vi "Test_of_the_stim_settings_save.vi"() -> ()   [LabVIEW 2016]
panel:
  out "Array 3":T1(array[cluster])
  out "Array 2":string[](array[string])
  out "data string 2":string
  out "value":T2(array[cluster])
  out "data string":string
  out "Array":T2(array[cluster])
  in  "Path to the settings file":path=path "D:/Users/Dmitriy/CData/CloudStation/Tracker_repository/Tracker_settings.tcf"
  in  "Stimulus presets":T1(array[cluster])=[{"Event type"=0, "Cond., s"=0.10000000149011612, "Stim., s"=0.10000000149011612, "Set/Clear"=FALSE, "TTL out N"=1, "Stim. has been set"=TRUE}, {"Event type"=0, "Cond., s"=0.20000000298023224, "Stim., s"=0.20000000298023224, "Set/Clear"=FALSE, "TTL out N"=2, "Stim. has been set"=TRUE}, {"Event type"=0, "Cond., s"=0.0, "Stim., s"=0.0, "Set/Clear"=FALSE, "TTL out N"=1, "Stim. has been set"=FALSE}, {"Event type"=0, "Cond., s"=0.4000000059604645, "Stim., s"=0.4000000059604645, "Set/Clear"=FALSE, "TTL out N"=2, "Stim. has been set"=TRUE}, {"Event type"=0, "Cond., s"=0.0, "Stim., s"=0.0, "Set/Clear"=FALSE, "TTL out N"=1, "Stim. has been set"=FALSE}, {"Event type"=0, "Cond., s"=0.0, "Stim., s"=0.0, "Set/Clear"=FALSE, "TTL out N"=1, "Stim. has been set"=FALSE}, {"Event type"=0, "Cond., s"=0.0, "Stim., s"=0.0, "Set/Clear"=FALSE, "TTL out N"=1, "Stim. has been set"=FALSE}, {"Event type"=0, "Cond., s"=0.0, "Stim., s"=0.0, "Set/Clear"=FALSE, "TTL out N"=1, "Stim. has been set"=FALSE}, {"Event type"=0, "Cond., s"=0.0, "Stim., s"=0.0, "Set/Clear"=FALSE, "TTL out N"=1, "Stim. has been set"=FALSE}, {"Event type"=0, "Cond., s"=0.0, "Stim., s"=0.0, "Set/Clear"=FALSE, "TTL out N"=1, "Stim. has been set"=FALSE}, {"Event type"=0, "Cond., s"=0.0, "Stim., s"=0.0, "Set/Clear"=FALSE, "TTL out N"=1, "Stim. has been set"=FALSE}, {"Event type"=0, "Cond., s"=0.0, "Stim., s"=0.0, "Set/Clear"=FALSE, "TTL out N"=1, "Stim. has been set"=FALSE}, {"Event type"=0, "Cond., s"=0.0, "Stim., s"=0.0, "Set/Clear"=FALSE, "TTL out N"=1, "Stim. has been set"=FALSE}, {"Event type"=0, "Cond., s"=0.0, "Stim., s"=0.0, "Set/Clear"=FALSE, "TTL out N"=1, "Stim. has been set"=FALSE}] {"TTL out N" items=["1"=1, "2"=2]; "Stim., s" min=0.0 max=10000.0 step=0.05000000074505806; "Cond., s" min=0.0 max=10000.0 step=0.05000000074505806 format="%#.2f"; "Event type" items=["Stay for N seconds"]}
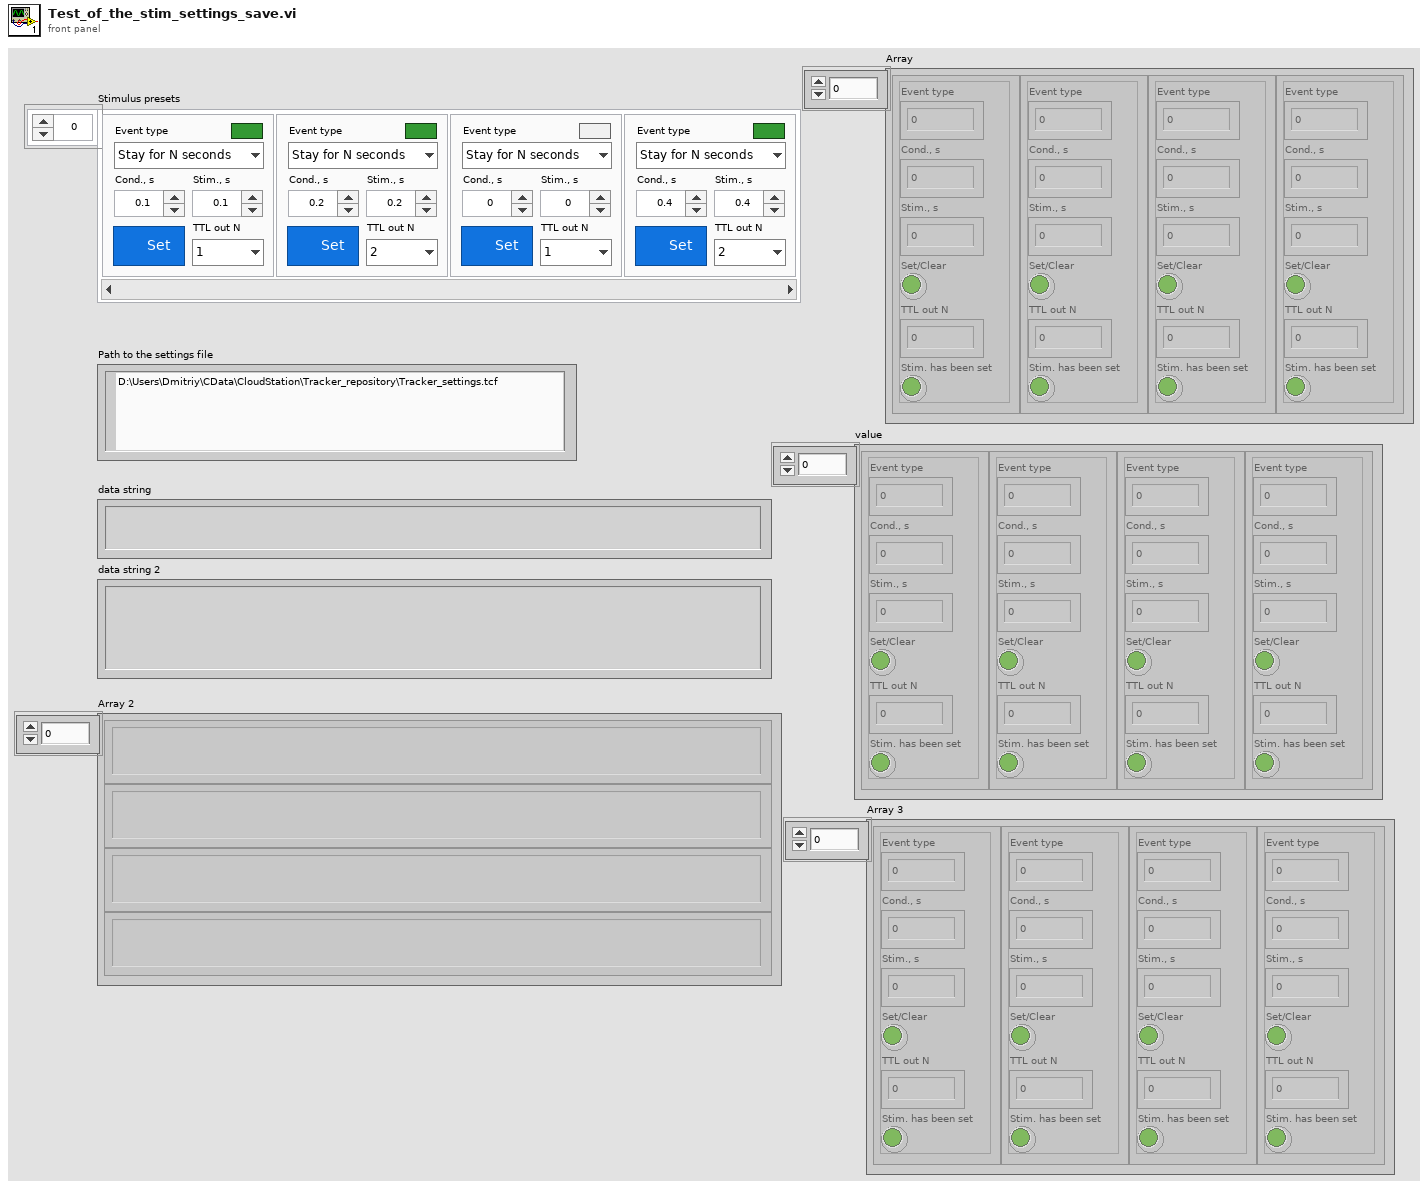
[diagram p1: front panel]
types:
  T1 = cluster{"Event type":u16, "Cond., s":dbl, "Stim., s":dbl, "Set/Clear":bool, "TTL out N":u16, "Stim. has been set":bool}[]
  T2 = cluster{"Event type":u16, "Cond., s":sgl, "Stim., s":sgl, "Set/Clear":bool, "TTL out N":u16, "Stim. has been set":bool}[]
  T3 = cluster{"Event type":u16, "Cond., s":dbl, "Stim., s":dbl, "Set/Clear":bool, "TTL out N":u16, "Stim. has been set":bool}
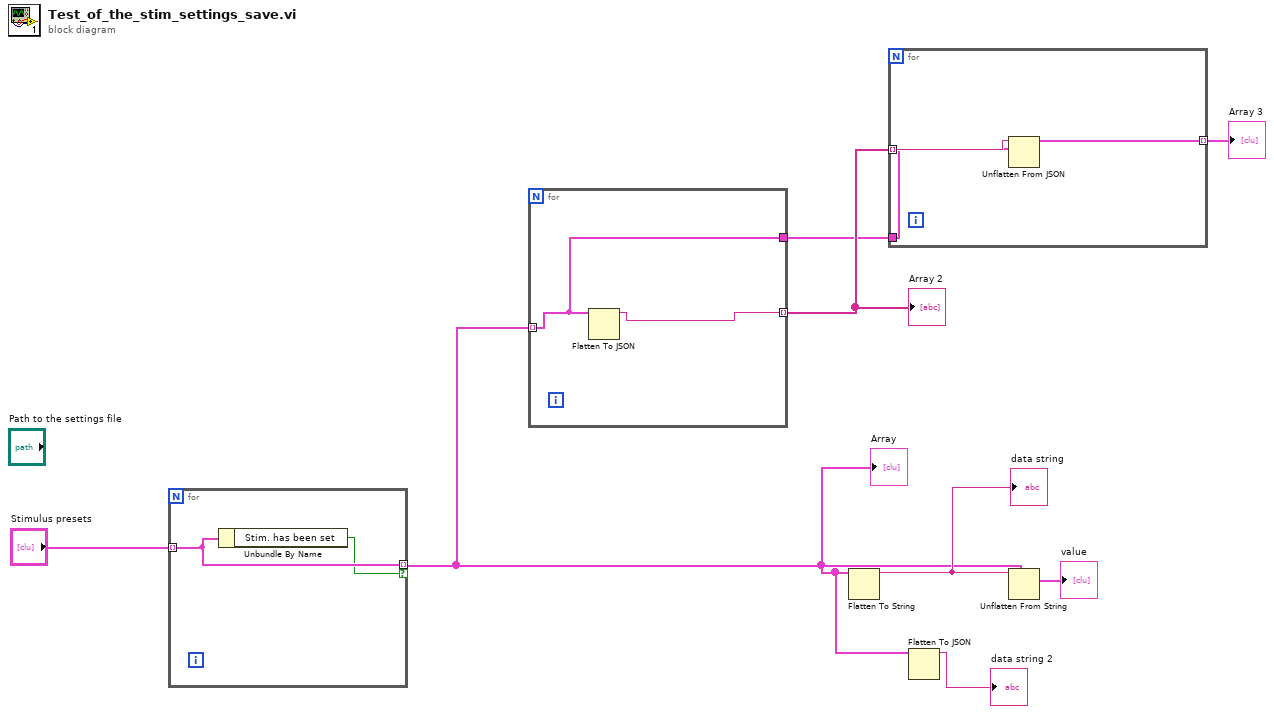
[diagram p0: block diagram]
diagram:
  n1 = for {
    tunnel: "Stimulus presets" -> [w10] mode=indexing
    tunnel: [w10] -> w4 mode=indexing if=w9
    n2 = Unbundle By Name(w10) -> ("Stim. has been set"=w9:bool)
  }
  "Array" <- w4
  n3 = for {
    tunnel: w4 -> [w11] mode=indexing
    tunnel: [w12] -> w3 mode=indexing
    tunnel: [w11] -> w2
    n4 = Flatten To JSON(anything=w11) -> (JSON string=w12:string)  [unwired: 2 in, 1 out]
  }
  "Array 2" <- w3
  n5 = Flatten To String(anything=w4) -> (data string=w7:string)  [unwired: 3 in, 2 out]
  "data string" <- w7
  n6 = for {
    tunnel: w3 -> [w15] mode=indexing
    tunnel: w2 -> [w14]
    tunnel: [w13] -> w1 mode=indexing
    n7 = Unflatten From JSON(JSON string=w15, type and defaults=w14) -> (value=w13:T3)  [unwired: 5 in, 1 out]
  }
  "Array 3" <- w1
  n8 = Flatten To JSON(anything=w4) -> (JSON string=→"data string 2":string)  [unwired: 2 in, 1 out]
  n9 = Unflatten From String(type=w4, binary string=w7) -> (value=→"value":T1)  [unwired: 3 in, 2 out]
